vi "Test Airmax.vi"() -> ()   [LabVIEW 2014, in "Airmar WS.lvclass"]
uses:
  Airmar WS.lvclass
  Data/Airmar Data.lvclass
  Reusable/Session APIs/Serial/Serial Session.lvclass
  Data/Airmar Data.lvclass/Airmar Data.ctl
  Airmar WS.lvclass/Airmar WS.ctl
  Data/Accessors/Read GGA.vi
  Data/Accessors/Read MDA.vi
  <userlib>/_Session Fwk/Session - Root.lvclass
panel:
  in  "change":bool
  out "MDA":T1
  out "GGA":T2
  out "error out":errorcluster
  in  "time":i16=10
  in  "Enable?":bool
  in  "CMD":string
  in  "Boolean":bool
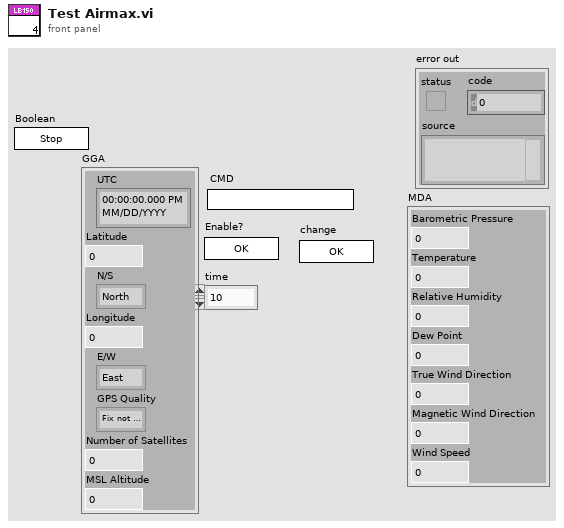
[diagram p1: front panel]
types:
  T1 = cluster{"Barometric Pressure":dbl, "Temperature":dbl, "Relative Humidity":dbl, "Dew Point":dbl, "True Wind Direction":dbl, "Magnetic Wind Direction":dbl, "Wind Speed":dbl}
  T2 = cluster{"UTC":timestamp, "Latitude":dbl, "N/S":enum8{"North", "South"}, "Longitude":dbl, "E/W":enum8{"East", "West"}, "GPS Quality":enum16{"Fix not available or invalid", "GPS SPS Mode, fix valid", "Differential GPS, SPS Mode, fix valid", "GPS PPS Mode, fix valid", "Real Time Kinematic", "Float RTK", "Estimated (dead reckoning) Mode", "Manual Input Mode", "Simulator Mode"}, "Number of Satellites":u8, "MSL Altitude":dbl}
  T3 = typedef "Session - Root.lvclass/Session Handle.ctl" = refnum<data-value>
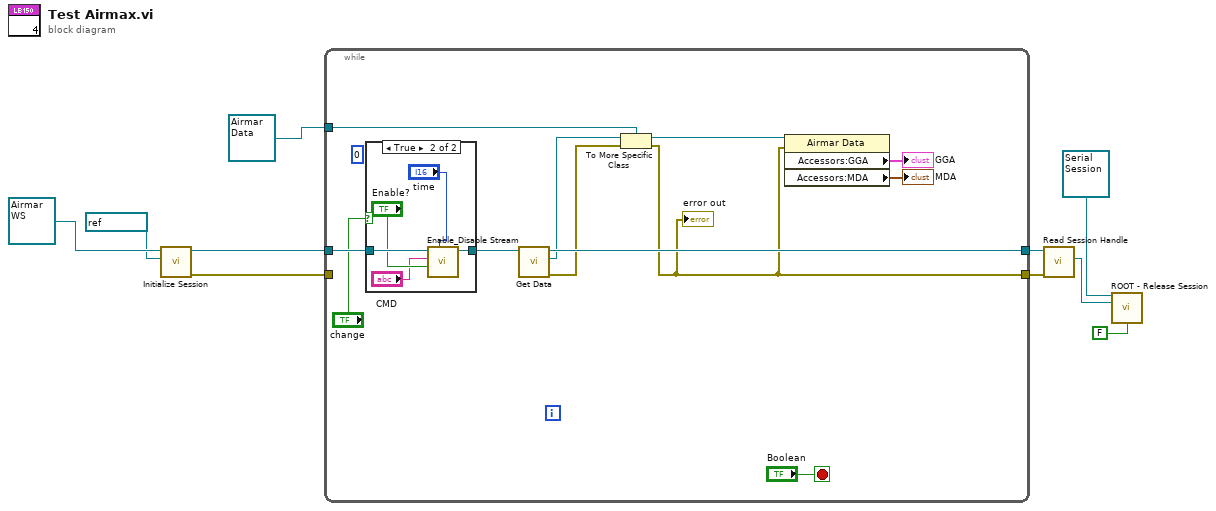
[diagram p0: block diagram]
diagram:
  n1 = call "Initialize Session.vi"("Port"=refnum<visa-resource-name> "COM5" ("VISA Resource"), "Airmar WS in"=refnum<class "Airmar WS.lvclass"> refnum) -> ("error out"=w1:errorcluster, "Airmar WS out"=w9:refnum<class "Airmar WS.lvclass">)  [unwired: 8 in]
  n2 = while {
    tunnel: w9 -> [w20]
    tunnel: [w22] -> w8
    tunnel: [w11] -> w6
    tunnel: refnum<class "Airmar Data.lvclass"> refnum ("Airmar Data") -> [w15]
    tunnel: w1 -> [_]
    stop <- "Boolean" stop-if-true
    (unwired) 0
    n3 = case shown="True" "change" {
      tunnel: w20 -> [w23 w28]
      tunnel: [w23 w27] -> w19
      frame False {
      }
      frame True {
        n4 = call "Enable_Disable Stream.vi"("time"="time", "Enable?"="Enable?", "String"="CMD", "Airmar WS in"=w28) -> ("Airmar WS out"=w27:refnum<class "Airmar WS.lvclass">)  [unwired: 6 in, 1 out]
      }
    }
    n5 = call-dynamic "Get Data.vi"("Airmar WS in"=w19) -> ("error out"=w12:errorcluster, "Data"=w14:refnum<class "Data.lvclass">, "Airmar WS out"=w22:refnum<class "Airmar WS.lvclass">)  [unwired: 8 in]
    n6 = To More Specific Class(target class=w15, reference=w14, error in=w12) -> (specific class reference=w13:refnum<class "Airmar Data.lvclass">, error out=w11:errorcluster)
    "error out" <- w11
    n7 = property class="Airmar Data"(reference=w13, error in=w11) -> ("Accessors:GGA"=→"GGA":T2, "Accessors:MDA"=→"MDA":T1)  [unwired: 2 out]
  }
  n8 = call "Read Session Handle.vi"("error in (no error)"=w6, "Airmar WS in"=w8) -> ("hSerial"=w5:T3)  [unwired: 7 in, 2 out]
  n9 = call <userlib>:"ROOT - Release Session.vi"("OBJ - Session in"=refnum<class "Serial Session.lvclass"> refnum ("Serial Session"), "Session Handle in"=w5, "force destroy? (F)"=FALSE) -> ()  [unwired: 10 in, 3 out]
